vi "SVL Exp Avg Level (resampled) (N Ch).vi"(6 "restart averaging (F)":bool, 8 "error in (no error)":errorcluster, 9 "exponential weighting":dbl=1.0 format="%.2f", 10 "even-angle channel info":T1[](array[typedef]) {"channel info"."pregain" format="%.2f"; "channel info"."weighting filter" items=["Linear", "A-weighting", "B-weighting", "C-weighting", "ITU-R 468-4", "Dolby", "CCITT", "C-message", "Wb", "Wc", "Wd", "We", "Wf", "Wh", "Wj", "Wk", "Wm", "AES17 20 kHz lowpass", "AES17 40 kHz lowpass", "AES17 20 kHz highpass", "AES17 40 kHz highpass"]; "channel info"."dB reference" format="%^.1e"; "channel info"."engineering units" items=["custom..."=0, "V"=1, "A"=21, "C"=30, "pC"=31, "s"=32, "-"=29, "Pa"=2, "N"=20, "g"=3, "m/s^2"=4, "m/s"=5, "m"=6, "mm/s"=12, "mm"=13, "micron/s"=14, "micron"=15, "in/s^2"=7, "in/s"=8, "in"=9, "mil/s"=10, "mil"=11, "rad/s^2"=16, "rad/s"=17, "rad"=18, "deg/s^2"=26, "deg/s"=27, "deg"=28, "RPM"=22, "cycle/s^2"=23, "Hz"=24, "cycle"=25, "strain"=19]; "channel info"."sensor sensitivity" format="%#_5f"}, 11 "even-angle signals [EU]":T5(array[cluster]) {"even-angle signal" format="%.2f"; "dr" format="%.2f"; "r0" format="%.2f"}) -> (0 "error out":errorcluster, 2 "unit labels":string[](array[string]), 3 "exp avg levels [EU rms]":cluster{"r0":dbl, "dr":dbl, "level":dbl[]}[](array[cluster]) {"level" format="%.2f"; "dr" format="%.2f"; "r0" format="%.2f"})   [LabVIEW 2017, in "SoundVib_VibrationLevel.lvlib"]
doc: "Computes the exponential averaged level of <B>scaled signal [EU]</B> or <B>even-angle signal [EU]</B>. <B>scaled signal [EU]</B> should have a zero DC component. You can attenuate the DC component with hardware AC-coupling filters and with software high-pass filters. Wire data to the <B>scaled signal [EU]</B> input to determine the polymorphic instance to use or manually select the instance."
uses:
  <vilib>/addons/Sound and Vibration/svt_Level/SoundVib_VibrationLevel.lvlib
  <vilib>/addons/_NISVFA/_Shared subVIs/Controls/svc_Resampled Channel Info.ctl
  <vilib>/addons/_NISVFA/_Shared subVIs/Controls/svc_Channel Info.ctl
  <vilib>/addons/_NISVFA/_Shared subVIs/Controls/svc_Engineering Units Text Ring.ctl
  <vilib>/addons/_NISVFA/_Shared subVIs/Controls/svc_Weighting Filter Text Ring.ctl
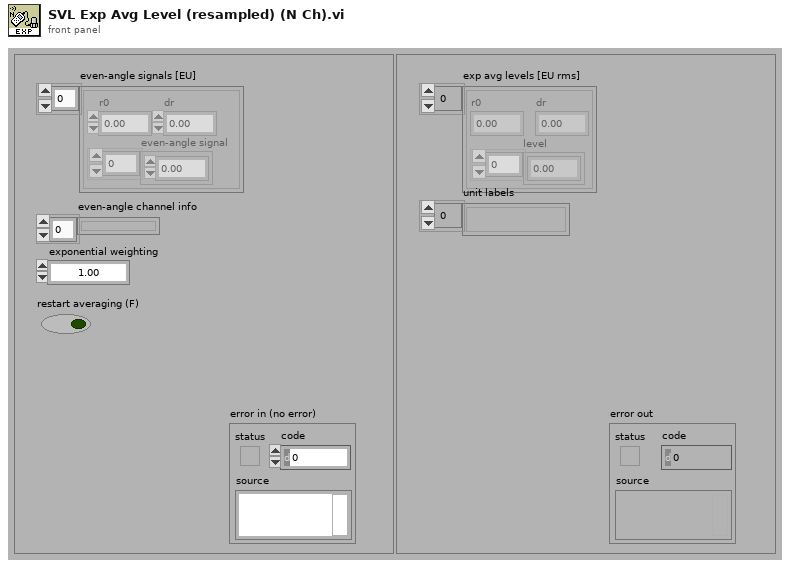
[diagram p1: front panel]
types:
  T1 = typedef "svc_Resampled Channel Info.ctl" = cluster{"channel name":string, "description":string, " channel info":T2}
  T2 = typedef "svc_Channel Info.ctl" = cluster{"sensor sensitivity":dbl, "engineering units":T3, "dB reference":dbl, "custom label":string, "weighting filter":T4, "pregain":dbl}
  T3 = typedef "svc_Engineering Units Text Ring.ctl" = u16
  T4 = typedef "svc_Weighting Filter Text Ring.ctl" = u16
  T5 = cluster{"r0":dbl, "dr":dbl, "even-angle signal":dbl[]}[]
  T6 = enum16{"RMS", "Running RMS", "Exp avg  ", "Dec exp avg ", "Peak", "Crest"}
  T7 = cluster{"r0":dbl, "dr":dbl, "even angle signal":dbl[]}[]
  T8 = enum16{"Reset filter", "Restart averaging", "Continue processing"}
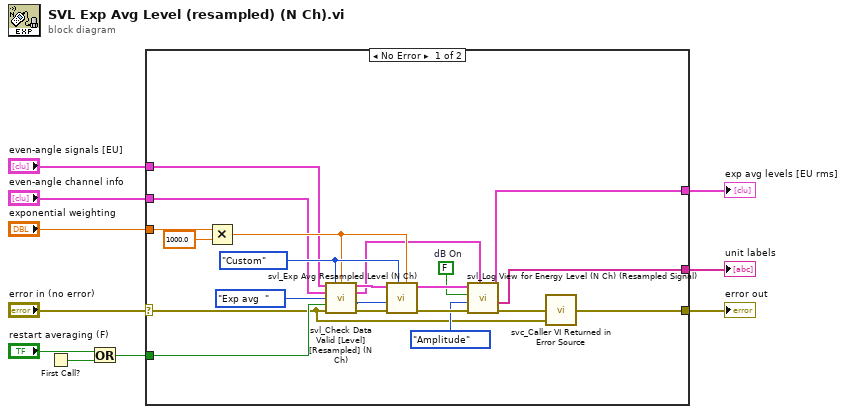
[diagram p0: block diagram]
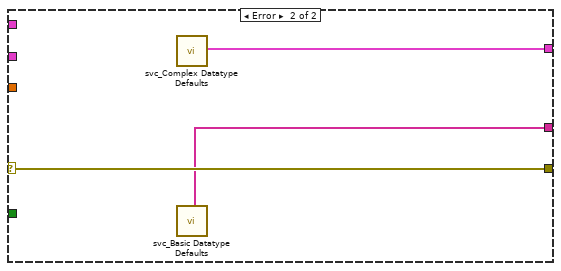
[diagram p2: hidden frame]
diagram:
  n1 = First Call?() -> (First Call?: T/F=w9:bool)
  n2 = Or(x="restart averaging (F)", y=w9) -> (x .or. y?=w8:bool)
  n3 = case shown="No Error" "error in (no error)" {
    selector: "error in (no error)" -> [w11 w34]
    tunnel: w8 -> [w22 _]
    tunnel: "even-angle signals [EU]" -> [w15 _]
    tunnel: [w14 w32] -> w6
    tunnel: [w23 w34] -> w5
    tunnel: [w25 w33] -> w4
    tunnel: "exponential weighting" -> [w18 _]
    tunnel: "even-angle channel info" -> [w13 _]
    frame No Error {
      w20 = enum16{"Slow", "Fast", "Impulse", "Custom"}."Custom" ("exponential mode")
      w28 = FALSE  # dB On
      n4 = Multiply(x=w18, y=1000.0 ("time constant [ms]")) -> (x*y=w17:dbl)
      n5 = call <vilib>:"svl_Check Data Valid [Level] [Resampled] (N Ch).vi"("scaled even angle signals [EU]"=w15, "exponential mode"=w20, "time constant [ms]"=w17, "even angle channel info"=w13, "level analysis"=T6."Exp avg  " ("Level Analysis"), "restart averaging (F)"=w22, "error in (no error)"=w11) -> ("dup scaled even angle signals [EU]"=w16:T7, "dup even angle channel info"=w12:T1[], "processing state"=w24:T8, "error out"=w31:errorcluster)  [unwired: 5 in]
      n6 = call <vilib>:"svl_Exp Avg Resampled Level (N Ch).vi"("timeConstant"=w17, "exponential mode"=w20, "error in (no error)"=w31, "processing state"=w24, "scaled signals"=w16) -> ("error out"=w30:errorcluster, "exp avg signals"=w29:T7)  [unwired: 3 in, 2 out]
      n7 = call <vilib>:"svl_Log View for Energy Level (N Ch) (Resampled Signal).vi"("even angle channel info"=w12, "error in (no error)"=w30, "view mode"=enum16{"Power", "Amplitude"}."Amplitude", "dB On (T)"=w28, "scaled even angle signals"=w29) -> ("error out"=w26:errorcluster, "unit labels"=w25:string[], "scaled even angle signals"=w14:T7)  [unwired: 4 in]
      n8 = call <vilib>:"svc_Caller VI Returned in Error Source.vi"("warning input to caller"=w11, "error in (no error)"=w26) -> ("error out"=w23:errorcluster)  [unwired: 3 in]
    }
    frame Error {
      n9 = call <vilib>:"svc_Complex Datatype Defaults.vi"() -> ("empty array of spectra"=w32:cluster{"f0":dbl, "df":dbl, "magnitude":dbl[]}[])  [unwired: 11 in, 8 out]
      n10 = call <vilib>:"svc_Basic Datatype Defaults.vi"() -> ("empty array of strings"=w33:string[])  [unwired: 7 in, 12 out]
    }
  }
  "exp avg levels [EU rms]" <- w6
  "unit labels" <- w4
  "error out" <- w5
